vi "Get CompactSubObj.vi"(8 "error in":errorcluster, 11 "DOMAIN in":refnum<class "DOMAIN.lvclass">) -> (0 "error out":errorcluster, 1 "Set?":bool, 2 "CompactSubObj":u8, 3 "DOMAIN out":refnum<class "DOMAIN.lvclass">)   [LabVIEW 2024, in "EDS.lvlib" / "DOMAIN.lvclass"]
uses:
  DOMAIN.lvclass
  D:/git/EDS-File-Viewer/Core/Object Type/Object Type Base.lvclass
  Object Type/Object Type Base.lvclass
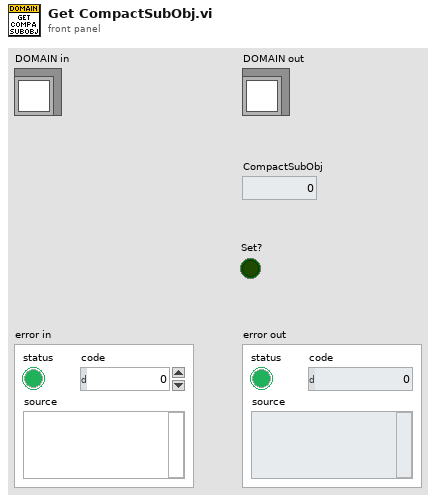
[diagram p1: front panel]
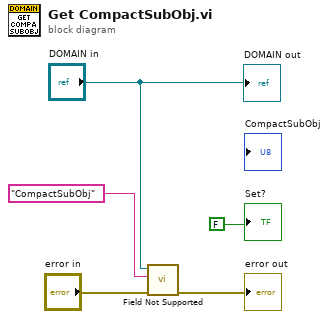
[diagram p0: block diagram]
diagram:
  n1 = call "Field Not Supported.vi"("error in"="error in", "Field name"="CompactSubObj", "Object Type in"="DOMAIN in") -> ("error out"=→"error out":errorcluster)  [unwired: 8 in]
  "DOMAIN out" <- "DOMAIN in"
  "Set?" <- FALSE ("Set?")
